vi "main.vi"() -> ()   [LabVIEW 2018]
doc: "This example demonstrates the use of binary morphological reconstruction in the particle analysis. The example allows you to keep the particles completely inside the ROI, completely outside the ROI or on the ROI."
uses:
  <vilib>/vision/NI_Vision_Development_Module.lvlib
panel:
  out "ROI左上角坐标":cluster{i32, i32}
  out "透射图灰度表":u32[](graph)
  out "反射图灰度表":u32[](graph)
  out "反射图":T1(plugin-control)
  in  "Font, Size & Style 3":T2={"Desired Font (Application)"=enum."Application Font", "[User-specified Font]"={"Font Name"="", "Size"=12, "Strikeout?"=FALSE, "Italic?"=FALSE, "Underline?"=FALSE, "Outline?"=FALSE, "Shadow?"=FALSE, "Bold?"=FALSE, "Rotation Angle"=0.0}, "Horizontal Alignment"=0, "Vertical Alignment"=0} {"Vertical Alignment" items=["Bottom", "Top", "Baseline"]; "Horizontal Alignment" items=["Left", "Center", "Right"]; "[User-specified Font]"."Rotation Angle" format="%.2f"}
  out "最大灰度值":sgl
  out "全图灰度级信息":T3 {"标准差" format="%.2f"; "均值" format="%.2f"; "相邻灰度级间隔" format="%.2f"; "起始灰度值" format="%.2f"; "最大值" format="%.2f"; "最小值" format="%.2f"}
  out "最大灰度值":sgl
  in  "预处理":bool
  in  "查看标注":bool
  in  "导入图像":bool
  in  "删除标注":bool
  in  "退出":bool
  out "标注框总数":dbl
  out "全图灰度级信息":T3 {"标准差" format="%.2f"; "均值" format="%.2f"; "相邻灰度级间隔" format="%.2f"; "起始灰度值" format="%.2f"; "最大值" format="%.2f"; "最小值" format="%.2f"}
  in  "Font, Size & Style 2":T2={"Desired Font (Application)"=enum."Application Font", "[User-specified Font]"={"Font Name"="", "Size"=12, "Strikeout?"=FALSE, "Italic?"=FALSE, "Underline?"=FALSE, "Outline?"=FALSE, "Shadow?"=FALSE, "Bold?"=FALSE, "Rotation Angle"=0.0}, "Horizontal Alignment"=0, "Vertical Alignment"=0} {"Vertical Alignment" items=["Bottom", "Top", "Baseline"]; "Horizontal Alignment" items=["Left", "Center", "Right"]; "[User-specified Font]"."Rotation Angle" format="%.2f"}
  in  "Font, Size & Style":T2={"Desired Font (Application)"=enum."Application Font", "[User-specified Font]"={"Font Name"="", "Size"=12, "Strikeout?"=FALSE, "Italic?"=FALSE, "Underline?"=FALSE, "Outline?"=FALSE, "Shadow?"=FALSE, "Bold?"=FALSE, "Rotation Angle"=0.0}, "Horizontal Alignment"=0, "Vertical Alignment"=0} {"Vertical Alignment" items=["Bottom", "Top", "Baseline"]; "Horizontal Alignment" items=["Left", "Center", "Right"]; "[User-specified Font]"."Rotation Angle" format="%.2f"}
  out "框组":T4(array[cluster])
  in  "Operation":enum16{"overlay rectangle"}(ring)
  out "标注图":T1(plugin-control)
  # "穿透法图像"
  # "反射法图像"
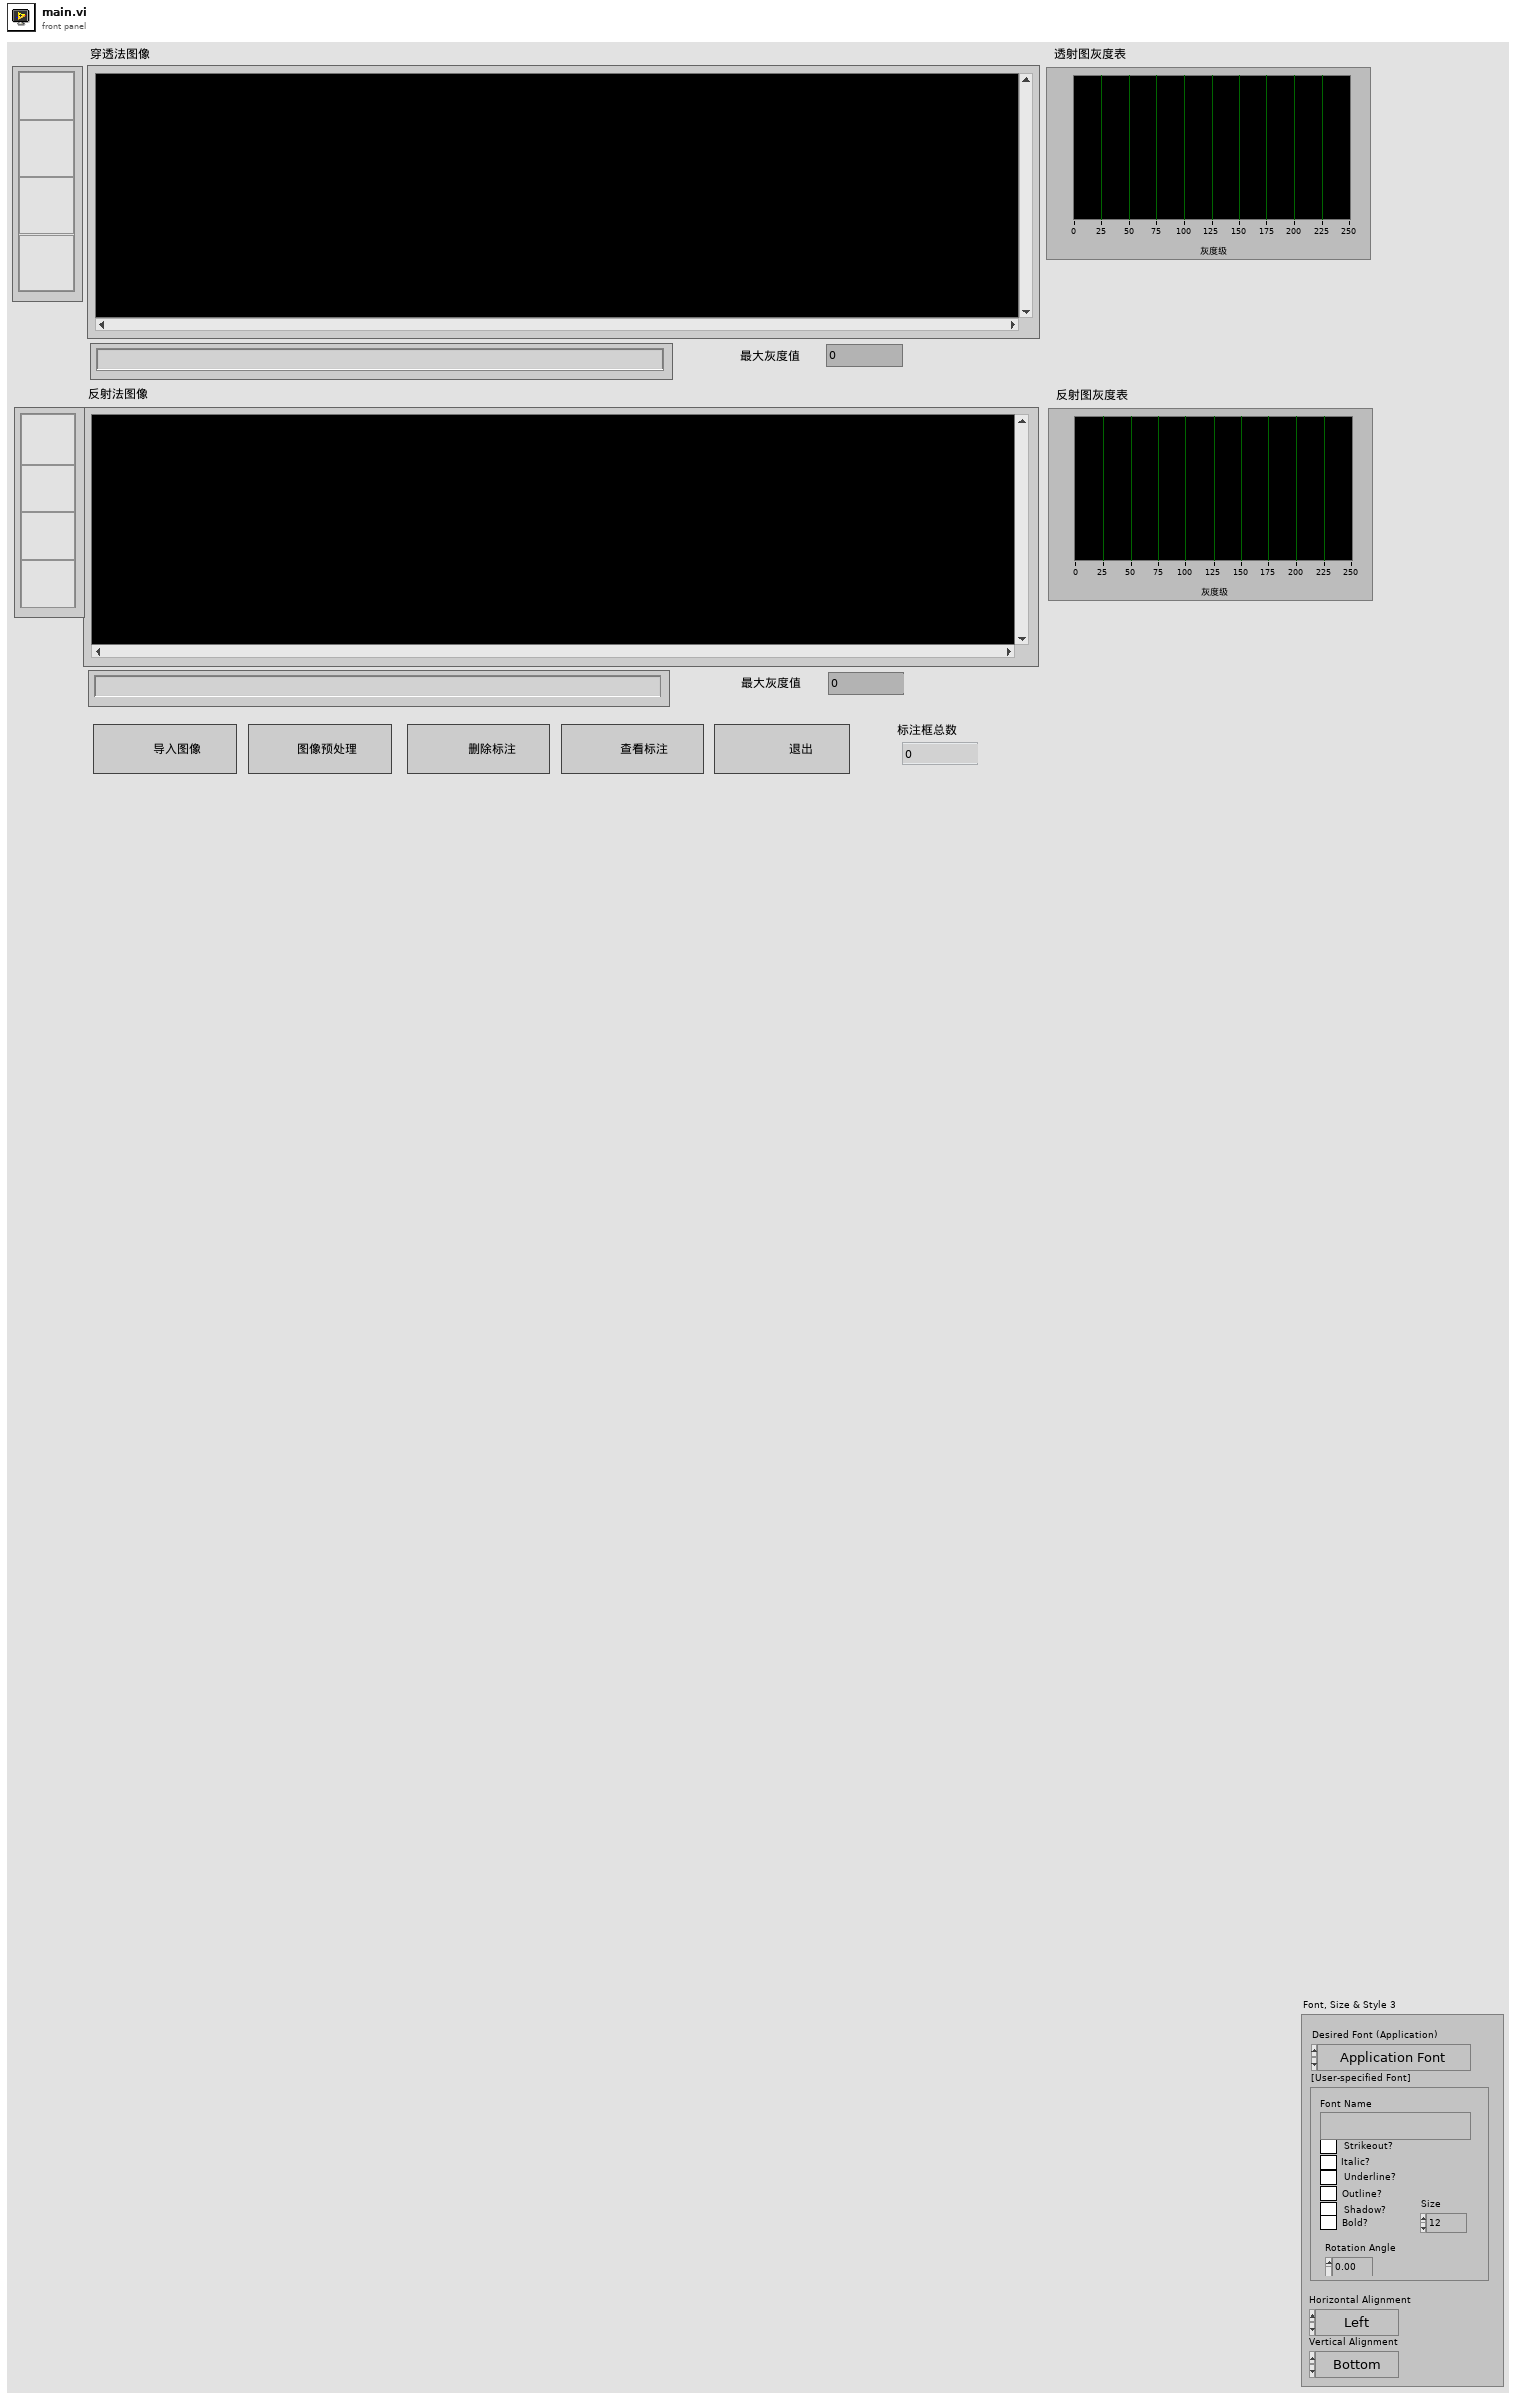
[diagram p1: front panel]
types:
  T1 = typedef "IMAQ Image.ctl" = refnum<image>
  T2 = cluster{"Desired Font (Application)":enum16{"User-specified Font", "Application Font", "System Font", "Dialog Font"}, "[User-specified Font]":cluster{"Font Name":string, "Size":i16, "Strikeout?":bool, "Italic?":bool, "Underline?":bool, "Outline?":bool, "Shadow?":bool, "Bold?":bool, "Rotation Angle":dbl}, "Horizontal Alignment":i16, "Vertical Alignment":i16}
  T3 = cluster{"histogram":u32[], "最小值":sgl, "最大值":sgl, "起始灰度值":sgl, "相邻灰度级间隔":sgl, "均值":sgl, "标准差":sgl, "像素面积":i32}
  T4 = cluster{"Global Rectangle":i32[], "Contours":cluster{"Contour Type":u32, "ROI Type":u32, "Points":i32[]}[]}[]
  T5 = typedef "Image Type" = u32
  T6 = cluster{"Global Rectangle":i32[], "Contours":cluster{"Contour Type":u32, "ROI Type":u32, "Points":i32[]}[]}
  T7 = cluster{"histogram":u32[], "Minimal Value":sgl, "Maximal Value":sgl, "Starting Value":sgl, "Interval Width":sgl, "Mean Value":sgl, "Standard  Variation":sgl, "Area (pixels)":i32}
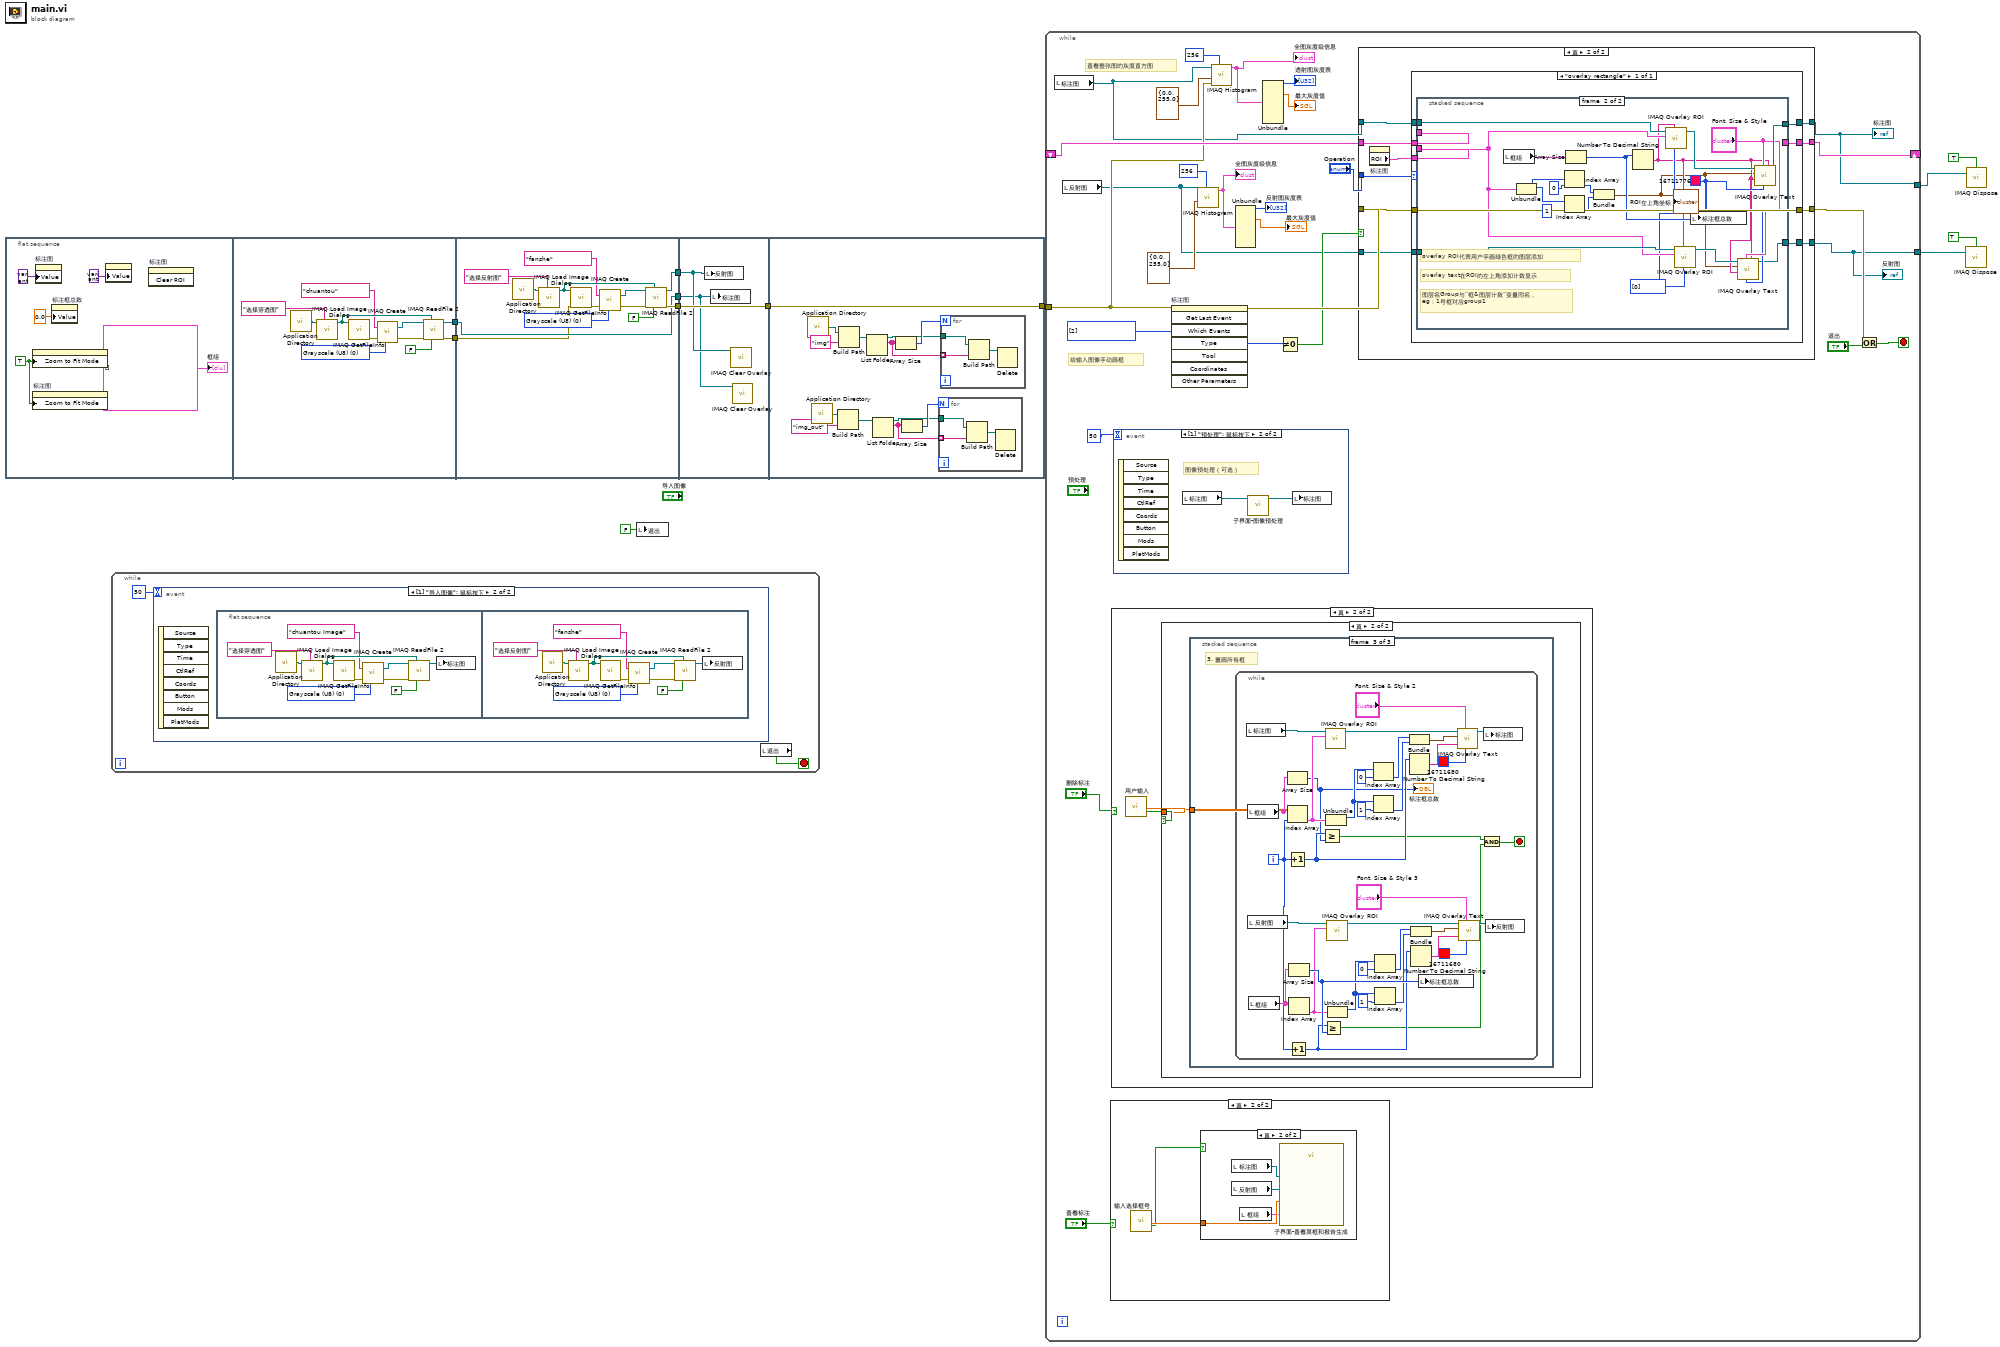
[diagram p0: block diagram]
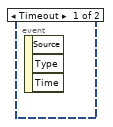
[diagram p2: hidden frame]
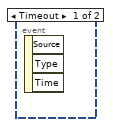
[diagram p3: hidden frame]
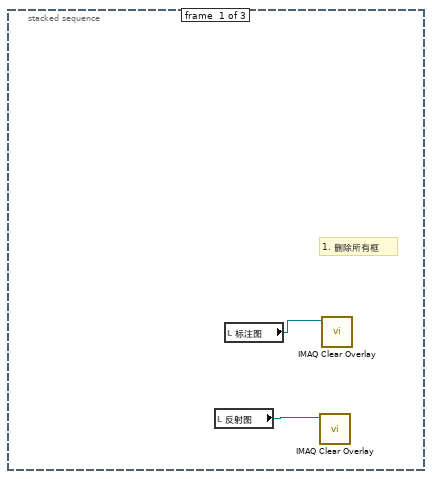
[diagram p8: hidden frame]
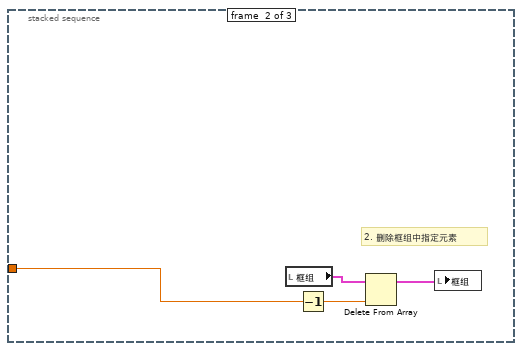
[diagram p9: hidden frame]
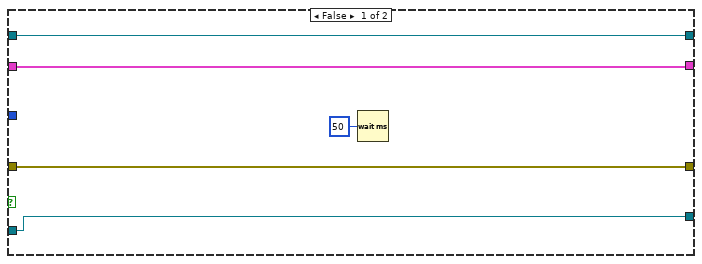
[diagram p10: hidden frame]
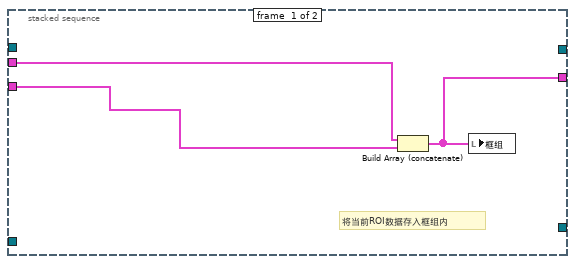
[diagram p11: hidden frame]
diagram:
  n1 = flat-sequence {
    tunnel: [w19] -> w9
    tunnel: [w18] -> w8
    tunnel: w9 -> [w30]
    tunnel: w8 -> [w31]
    tunnel: [w32] -> w7
    tunnel: [w31] -> w6
    tunnel: [w29] -> w5
    tunnel: w7 -> [w44]
    tunnel: w6 -> [w42]
    tunnel: w5 -> [w43]
    tunnel: [w44] -> w1
    tunnel: [w57] -> w12
    tunnel: w1 -> [w57]
    frame #0 {
      w16 = TRUE ("Zoom to Fit Mode")
      n2 = property on="反射图" class="ImageControl"("Zoom to Fit Mode"=w16) -> ()  [unwired: 2 in, 2 out]
      n3 = property on="标注图" class="ImageControl"("Zoom to Fit Mode"=w16) -> ()  [unwired: 2 in, 2 out]
      n4 = property on="标注图" class="ImageControl"("Value"=variant ("值")) -> ()  [unwired: 2 in, 2 out]
      n5 = property on="标注框总数" class="DigNum (严格)"("Value"=0.0 ("标注框总数")) -> ()  [unwired: 2 in, 2 out]
      n6 = property on="反射图" class="ImageControl"("Value"=variant ("值")) -> ()  [unwired: 2 in, 2 out]
      n7 = invoke on="标注图" class="ImageControl" method="Clear ROI"() -> ()  [unwired: 3 in, 3 out]
      "框组" <- T4 [] ("框组")
    }
    frame #1 {
      w20 = T5 0 items=["Grayscale (U8)", "Grayscale (I16)", "Grayscale (SGL)", "Complex (CSG)", "RGB (U32)", "HSL (U32)", "RGB (U64)", "Grayscale (U16)"] ("Image Type")
      n8 = call <vilib>:"Application Directory.vi"() -> ("Application Directory"=w28:path)
      n9 = call "IMAQ Load Image Dialog"("Prompt"="选择穿透图" ("prompt"), "Start Path"=w28) -> ("Path"=w24:path)  [unwired: 7 in, 2 out]
      n10 = call "IMAQ GetFileInfo"("File Path"=w24) -> ("error out"=w25:errorcluster)  [unwired: 4 in, 6 out]
      n11 = call "IMAQ Create"("Image Name"="chuantou", "Image Type"=w20, "error in (no error)"=w25) -> ("New Image"=w26:T1, "error out"=w27:errorcluster)  [unwired: 2 in]
      n12 = call "IMAQ ReadFile 2"("Use File Path Image Type"=FALSE, "File Path"=w24, "error in (no error)"=w27, "Image"=w26) -> ("error out"=w19:errorcluster, "Image Out"=w18:T1)  [unwired: 3 in, 3 out]
    }
    frame #2 {
      w33 = T5 0 items=["Grayscale (U8)", "Grayscale (I16)", "Grayscale (SGL)", "Complex (CSG)", "RGB (U32)", "HSL (U32)", "RGB (U64)", "Grayscale (U16)"] ("Image Type")
      n13 = call <vilib>:"Application Directory.vi"() -> ("Application Directory"=w41:path)
      n14 = call "IMAQ Load Image Dialog"("Prompt"="选择反射图" ("prompt"), "Start Path"=w41) -> ("Path"=w37:path)  [unwired: 7 in, 2 out]
      n15 = call "IMAQ GetFileInfo"("error in (no error)"=w30, "File Path"=w37) -> ("error out"=w38:errorcluster)  [unwired: 3 in, 6 out]
      n16 = call "IMAQ Create"("Image Name"="fanshe", "Image Type"=w33, "error in (no error)"=w38) -> ("New Image"=w39:T1, "error out"=w40:errorcluster)  [unwired: 2 in]
      n17 = call "IMAQ ReadFile 2"("Use File Path Image Type"=FALSE, "File Path"=w37, "error in (no error)"=w40, "Image"=w39) -> ("error out"=w32:errorcluster, "Image Out"=w29:T1)  [unwired: 3 in, 3 out]
    }
    frame #3 {
      n18 = local write "反射图"(w43) -> ()
      n19 = local write "标注图"(w42) -> ()
      n20 = call "IMAQ Clear Overlay"("Image"=w43) -> ()  [unwired: 9 in, 2 out]
      n21 = call "IMAQ Clear Overlay"("Image"=w42) -> ()  [unwired: 9 in, 2 out]
    }
    frame #4 {
      n22 = call <vilib>:"Application Directory.vi"() -> ("Application Directory"=w53:path)
      n23 = call <vilib>:"Application Directory.vi"() -> ("Application Directory"=w47:path)
      n24 = Build Path(base path=w47, name or relative path="img_out" ("名称或相对路径")) -> (appended path=w48:path)
      n25 = Build Path(base path=w53, name or relative path="img" ("名称或相对路径")) -> (appended path=w54:path)
      n26 = List Folder(path=w54) -> (path out=w52:path, filenames=w56:string[])  [unwired: 3 in, 2 out]
      n27 = List Folder(path=w48) -> (path out=w46:path, filenames=w50:string[])  [unwired: 3 in, 2 out]
      n28 = Array Size(array=w56) -> (size(s)=w55:i32)
      n29 = Array Size(array=w50) -> (size(s)=w49:i32)
      n30 = for {
        N: w49 -> [_]
        tunnel: w46 -> [w59]
        tunnel: w50 -> [w58] mode=indexing
        n31 = Build Path(base path=w59, name or relative path=w58) -> (appended path=w60:path)
        n32 = Delete(path (use dialog)=w60) -> ()  [unwired: 4 in, 3 out]
      }
      n33 = for {
        N: w55 -> [_]
        tunnel: w52 -> [w62]
        tunnel: w56 -> [w61] mode=indexing
        n34 = Build Path(base path=w62, name or relative path=w61) -> (appended path=w63:path)
        n35 = Delete(path (use dialog)=w63) -> ()  [unwired: 4 in, 3 out]
      }
    }
  }
  n36 = while {
    stop <- w64 stop-if-true
    n37 = event shown="[1] \"导入图像\": 鼠标按下" {
      selector: _ -> [_ _]
      dyn-events: _ -> [_ _]
      timeout: 50 -> [_ _]
      event Timeout {
        n38 = event-data() -> ()  [unwired: 1 in, 3 out]
      }
      event "导入图像": Mouse Down {
        n39 = event-data() -> ()  [unwired: 1 in, 8 out]
        n40 = flat-sequence {
          frame #0 {
            w67 = T5 0 items=["Grayscale (U8)", "Grayscale (I16)", "Grayscale (SGL)", "Complex (CSG)", "RGB (U32)", "HSL (U32)", "RGB (U64)", "Grayscale (U16)"] ("Image Type")
            n41 = call <vilib>:"Application Directory.vi"() -> ("Application Directory"=w75:path)
            n42 = call "IMAQ Load Image Dialog"("Prompt"="选择穿透图" ("prompt"), "Start Path"=w75) -> ("Path"=w71:path)  [unwired: 7 in, 2 out]
            n43 = call "IMAQ GetFileInfo"("File Path"=w71) -> ("error out"=w72:errorcluster)  [unwired: 4 in, 6 out]
            n44 = call "IMAQ Create"("Image Name"="chuantou Image", "Image Type"=w67, "error in (no error)"=w72) -> ("New Image"=w73:T1, "error out"=w74:errorcluster)  [unwired: 2 in]
            n45 = call "IMAQ ReadFile 2"("Use File Path Image Type"=FALSE, "File Path"=w71, "error in (no error)"=w74, "Image"=w73) -> ("Image Out"=w66:T1)  [unwired: 3 in, 4 out]
            n46 = local write "标注图"(w66) -> ()
          }
          frame #1 {
            w79 = T5 0 items=["Grayscale (U8)", "Grayscale (I16)", "Grayscale (SGL)", "Complex (CSG)", "RGB (U32)", "HSL (U32)", "RGB (U64)", "Grayscale (U16)"] ("Image Type")
            n47 = call <vilib>:"Application Directory.vi"() -> ("Application Directory"=w81:path)
            n48 = call "IMAQ Load Image Dialog"("Prompt"="选择反射图" ("prompt"), "Start Path"=w81) -> ("Path"=w85:path)  [unwired: 7 in, 2 out]
            n49 = call "IMAQ GetFileInfo"("File Path"=w85) -> ("error out"=w84:errorcluster)  [unwired: 4 in, 6 out]
            n50 = call "IMAQ Create"("Image Name"="fanshe", "Image Type"=w79, "error in (no error)"=w84) -> ("New Image"=w83:T1, "error out"=w82:errorcluster)  [unwired: 2 in]
            n51 = call "IMAQ ReadFile 2"("Use File Path Image Type"=FALSE, "File Path"=w85, "error in (no error)"=w82, "Image"=w83) -> ("Image Out"=w76:T1)  [unwired: 3 in, 4 out]
            n52 = local write "反射图"(w76) -> ()
          }
        }
      }
    }
    n53 = local read "退出"() -> (w64:bool)
  }
  n54 = local write "退出"(FALSE ("退出")) -> ()
  n55 = while {
    shift-right: [w106] -> _
    shift-left: _ -> [w105]
    tunnel: w12 -> [w104]
    tunnel: [w88] -> w10
    tunnel: [w89] -> w3
    stop <- w108 stop-if-true
    w111 = i32[] [2] items=["No Event"=0, "Click Event"=1, "Draw Event"=2, "Size Event"=4, "Scroll Event"=5, "Double Click Event"=8] ("Which Events")
    # "给输入图像手动画框"
    # "查看整张图的灰度直方图"
    n56 = local read "标注图"() -> (w90:T1)
    n57 = local read "反射图"() -> (w91:T1)
    n58 = case shown="真" "查看标注" {
      frame False {
      }
      frame True {
        n59 = call "输入选择框号"() -> ("框号"=w117:dbl, "确定"=w116:bool)  [unwired: 17 in, 1 out]
        n60 = case shown="真" w116 {
          tunnel: w117 -> [_ w121]
          frame False {
            # "用户取消操作"
          }
          frame True {
            n61 = local read "标注图"() -> (w118:T1)
            n62 = local read "反射图"() -> (w119:T1)
            n63 = local read "框组"() -> (w120:T4)
            n64 = call "子界面-查看某框和报告生成.vi"("框号"=w121, "框组"=w120, "反射图"=w119, "标注图"=w118) -> ()  [unwired: 2 in]
          }
        }
      }
    }
    n65 = case shown="真" "删除标注" {
      frame False {
      }
      frame True {
        n66 = call "用户输入"() -> ("框号"=w122:dbl, "确定"=w123:bool)  [unwired: 17 in, 1 out]
        n67 = case shown="真" w123 {
          tunnel: w122 -> [_ w124]
          frame False {
            # "用户取消操作"
          }
          frame True {
            n68 = stacked-sequence {
              tunnel: w124 -> [_ w129 _]
              frame #0 {
                # "1. 删除所有框"
                n69 = local read "反射图"() -> (w125:T1)
                n70 = local read "标注图"() -> (w126:T1)
                n71 = call "IMAQ Clear Overlay"("Image"=w125) -> ()  [unwired: 9 in, 2 out]
                n72 = call "IMAQ Clear Overlay"("Image"=w126) -> ()  [unwired: 9 in, 2 out]
              }
              frame #1 {
                # "2. 删除框组中指定元素"
                n73 = local read "框组"() -> (w130:T4)
                n74 = Decrement(x=w129) -> (x-1=w128:dbl)
                n75 = Delete From Array(array=w130, index=w128) -> (array with subset deleted=w127:T4)  [unwired: 1 in, 1 out]
                n76 = local write "框组"(w127) -> ()
              }
              frame #2 {
                # "3. 重画所有框"
                n77 = while {
                  i -> [w134]
                  stop <- w131 stop-if-true
                  n78 = local read "标注图"() -> (w166:T1)
                  n79 = local read "框组"() -> (w160:T4)
                  n80 = local read "反射图"() -> (w135:T1)
                  n81 = local read "框组"() -> (w141:T4)
                  n82 = Array Size(array=w160) -> (size(s)=w151:i32)
                  "标注框总数" <- w151
                  n83 = Index Array(array=w160, index=w134) -> (element=w153:T6)
                  n84 = Increment(x=w134) -> (x+1=w165:i32)
                  n85 = Array Size(array=w141) -> (size(s)=w150:i32)
                  n86 = Index Array(array=w141) -> (element=w148:T6)  [unwired: 1 in]
                  n87 = Increment(x=w134) -> (x+1=w136:i32)
                  n88 = Greater Or Equal?(x=w165, y=w151) -> (x >= y?=w133:bool)
                  n89 = Greater Or Equal?(x=w136, y=w150) -> (x >= y?=w132:bool)
                  n90 = call "IMAQ Overlay ROI"("ROI Descriptor"=w153, "Image"=w166) -> ("Image Out"=w162:T1)  [unwired: 8 in, 1 out]
                  n91 = Unbundle(w153) -> ("Global Rectangle"=w156:i32[])  [unwired: 1 out]
                  n92 = call "IMAQ Overlay ROI"("ROI Descriptor"=w148, "Image"=w135) -> ("Image Out"=w139:T1)  [unwired: 8 in, 1 out]
                  n93 = Unbundle(w148) -> ("Global Rectangle"=w145:i32[])  [unwired: 1 out]
                  n94 = Index Array(array=w156, index=0 ("索引")) -> (element=w157:i32)
                  n95 = Index Array(array=w156, index=1 ("索引")) -> (element=w158:i32)
                  n96 = Index Array(array=w145, index=0 ("索引")) -> (element=w144:i32)
                  n97 = Index Array(array=w145, index=1 ("索引")) -> (element=w143:i32)
                  n98 = Bundle(w157, w158) -> (w155:cluster{i32, i32})  [unwired: 1 in]
                  n99 = Number To Decimal String(number=w165) -> (decimal integer string=w163:string)  [unwired: 1 in]
                  n100 = Bundle(w144, w143) -> (w146:cluster{i32, i32})  [unwired: 1 in]
                  n101 = Number To Decimal String(number=w136) -> (decimal integer string=w138:string)  [unwired: 1 in]
                  n102 = local write "标注框总数"(w150) -> ()
                  n103 = call "IMAQ Overlay Text"("Text Color (black)"=u32 16711680, "Font, Size & Style"="Font, Size & Style 2", "String"=w163, "Origin"=w155, "Image"=w162) -> ("Image Out"=w161:T1)  [unwired: 5 in, 1 out]
                  n104 = call "IMAQ Overlay Text"("Text Color (black)"=u32 16711680, "Font, Size & Style"="Font, Size & Style 3", "String"=w138, "Origin"=w146, "Image"=w139) -> ("Image Out"=w140:T1)  [unwired: 5 in, 1 out]
                  n105 = And(x=w133, y=w132) -> (x .and. y?=w131:bool)
                  n106 = local write "标注图"(w161) -> ()
                  n107 = local write "反射图"(w140) -> ()
                }
              }
            }
          }
        }
      }
    }
    n108 = event shown="[1] \"预处理\": 鼠标按下" {
      selector: _ -> [_ _]
      dyn-events: _ -> [_ _]
      timeout: 50 -> [_ _]
      event Timeout {
        n109 = event-data() -> ()  [unwired: 1 in, 3 out]
      }
      event "预处理": Mouse Down {
        # "图像预处理（可选）"
        n110 = event-data() -> ()  [unwired: 1 in, 8 out]
        n111 = local read "标注图"() -> (w115:T1)
        n112 = call "子界面-图像预处理.vi"("原图"=w115) -> ("处理后"=w114:T1)  [unwired: 10 in]
        n113 = local write "标注图"(w114) -> ()
      }
    }
    n114 = invoke on="标注图" class="ImageControl" method="Get Last Event"(error in=w104, "Which Events"=w111) -> (error out=w110:errorcluster, "Type"=w112:i32)  [unwired: 6 in, 6 out]
    n115 = call "IMAQ Histogram"("Number of Classes"=256, "Interval Range"=cluster{"Minimum":sgl, "Maximum":sgl} {"Minimum"=0.0, "Maximum"=255.0}, "Image"=w91) -> ("Histogram Report"=w93:T7)  [unwired: 7 in, 1 out]
    "全图灰度级信息" <- w93
    n116 = call "IMAQ Histogram"("Number of Classes"=256, "error in (no error)"=w104, "Interval Range"=cluster{"Minimum":sgl, "Maximum":sgl} {"Minimum"=0.0, "Maximum"=255.0}, "Image"=w90) -> ("Histogram Report"=w95:T7)  [unwired: 6 in, 1 out]
    "全图灰度级信息" <- w95
    n117 = Unbundle(w93) -> ("histogram"=→"反射图灰度表":u32[], "Maximal Value"=→"最大灰度值":sgl)  [unwired: 6 out]
    n118 = Unbundle(w95) -> ("histogram"=→"透射图灰度表":u32[], "Maximal Value"=→"最大灰度值":sgl)  [unwired: 6 out]
    n119 = Not Equal To 0?(x=w112) -> (x != 0?=w107:bool)
    n120 = case shown="真" w107 {
      tunnel: w90 -> [w171 w181]
      tunnel: [w171 w180] -> w88
      tunnel: "Operation" -> [_ w178]
      tunnel: w110 -> [w170 w177]
      tunnel: [w170 w176] -> w109
      tunnel: [w168 w175] -> w106
      tunnel: w105 -> [w168 w174]
      tunnel: w91 -> [w167 w173]
      tunnel: [w167 w172] -> w89
      frame False {
        n121 = Wait (ms)(milliseconds to wait=u32 50) -> ()  [unwired: 1 out]
      }
      frame True {
        n122 = property on="标注图" class="ImageControl"() -> ("ROI"=w179:T6)  [unwired: 2 in, 2 out]
        n123 = case shown="\"overlay rectangle\"" w178 {
          tunnel: w181 -> [w188]
          tunnel: w179 -> [w186]
          tunnel: [w187] -> w180
          tunnel: w177 -> [w189]
          tunnel: [w189] -> w176
          tunnel: [w185] -> w175
          tunnel: w174 -> [w184]
          tunnel: w173 -> [w183]
          tunnel: [w182] -> w172
          frame "overlay rectangle" {
            n124 = stacked-sequence {
              tunnel: w188 -> [_ w204]
              tunnel: [_ w203] -> w187
              tunnel: w186 -> [w192 w200]
              tunnel: [w190 _] -> w185
              tunnel: w184 -> [w191 _]
              tunnel: w183 -> [_ w201]
              tunnel: [_ w197] -> w182
              frame #0 {
                # "将当前ROI数据存入框组内"
                n125 = Build Array (concatenate)(w191, w192) -> (w190:T4)
                n126 = local write "框组"(w190) -> ()
              }
              frame #1 {
                w195 = u32[] [0] ("Colors (Green)")
                w198 = u32 16711776 ("Text Color (black)")
                # "图层名Group与“框&图层计数”变量同名，\neg：1号框对应group1"
                # "overlay text在ROI的左上角添加计数显示"
                # "overlay ROI代表用户手画绿色框的图层添加"
                n127 = local read "框组"() -> (w207:T4)
                n128 = Unbundle(w200) -> ("Global Rectangle"=w210:i32[])  [unwired: 1 out]
                n129 = Index Array(array=w210, index=0 ("索引")) -> (element=w209:i32)
                n130 = Index Array(array=w210, index=1 ("索引")) -> (element=w208:i32)
                n131 = Array Size(array=w207) -> (size(s)=w202:i32)
                n132 = Bundle(w209, w208) -> (w193:cluster{i32, i32})  [unwired: 1 in]
                "ROI左上角坐标" <- w193
                n133 = Number To Decimal String(number=w202) -> (decimal integer string=w194:string)  [unwired: 1 in]
                n134 = call "IMAQ Overlay ROI"("Colors (Green)"=w195, "Group"=w194, "ROI Descriptor"=w200, "Image"=w204) -> ("Image Out"=w211:T1)  [unwired: 6 in, 1 out]
                n135 = call "IMAQ Overlay ROI"("Colors (Green)"=w195, "Group"=w194, "ROI Descriptor"=w200, "Image"=w201) -> ("Image Out"=w196:T1)  [unwired: 6 in, 1 out]
                n136 = local write "标注框总数"(w202) -> ()
                n137 = call "IMAQ Overlay Text"("Group"=w194, "Text Color (black)"=w198, "Font, Size & Style"="Font, Size & Style", "String"=w194, "Origin"=w193, "Image"=w196) -> ("Image Out"=w197:T1)  [unwired: 4 in, 1 out]
                n138 = call "IMAQ Overlay Text"("Group"=w194, "Text Color (black)"=w198, "Font, Size & Style"="Font, Size & Style", "String"=w194, "Origin"=w193, "Image"=w211) -> ("Image Out"=w203:T1)  [unwired: 4 in, 1 out]
              }
            }
          }
        }
      }
    }
    "标注图" <- w88
    "反射图" <- w89
    n139 = Or(x=w109, y="退出") -> (x .or. y?=w108:bool)
  }
  n140 = call "IMAQ Dispose"("All Images? (No)"=TRUE, "Image"=w3) -> ()  [unwired: 1 in, 4 out]
  n141 = call "IMAQ Dispose"("All Images? (No)"=TRUE, "Image"=w10) -> ()  [unwired: 1 in, 4 out]
